vi "Next index.vi"(2 "size(s)":i32[](array[numeric]), 3 "Current Index":u32[](array[numeric])) -> (0 "last state":bool, 1 "Next Index":u32[](array[numeric]))   [LabVIEW 2012]
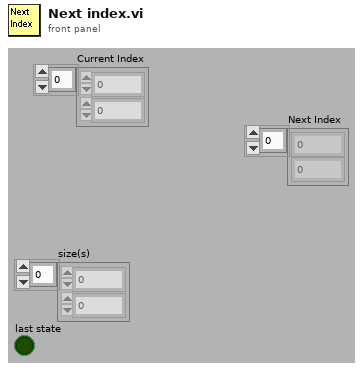
[diagram p1: front panel]
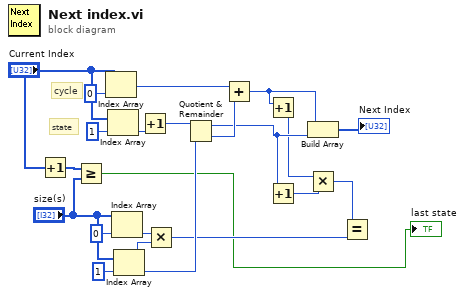
[diagram p0: block diagram]
diagram:
  # "state"
  # "cycle"
  n1 = Increment(x="Current Index") -> (x+1=w5:u32[])
  n2 = Greater Or Equal?(x=w5, y="size(s)") -> (x >= y?=→"last state":bool)
  n3 = Index Array(array="Current Index", index=0) -> (element=w14:u32)
  n4 = Index Array(array="Current Index", index=1) -> (element=w17:u32)
  n5 = Index Array(array="size(s)", index=0) -> (element=w8:i32)
  n6 = Index Array(array="size(s)", index=1) -> (element=w15:i32)
  n7 = Increment(x=w17) -> (x+1=w16:u32)
  n8 = Multiply(x=w8, y=w15) -> (x*y=w6:i32)
  n9 = Quotient & Remainder(x=w16, y=w15) -> (x-y*floor(x/y)=w12:u32, floor(x/y)=w13:u32)
  n10 = Add(x=w14, y=w13) -> (x+y=w11:u32)
  n11 = Increment(x=w11) -> (x+1=w10:u32)
  n12 = Increment(x=w12) -> (x+1=w9:u32)
  n13 = Build Array(w11, w12) -> (→"Next Index":u32[])
  n14 = Multiply(x=w10, y=w9) -> (x*y=w7:u32)
  n15 = Equal?(x=w7, y=w6) -> ()  [unwired: 1 out]
